vi "Final_Simulator_Run.vi"(7 "Mass Flow (lbm/min) vs. Pressure Drop (inH2O) - Real Data":dbl[][](array[numeric])=[[0.5, 0.015], [1.0, 0.062], [1.5, 0.141], [2.0, 0.252], [2.5, 0.395], [3.5, 0.778]], 8 "error in (no error)":errorcluster, 9 "Tuners":T1={"Inlet Diameter (in)"=0.0, "Outlet Diameter (in)"=0.0, " Length (in)"=0.0, "   Diameter (in)"=0.0, "D_h (in)"=0.0, "OAR"=0.95, "Run Optimizer"=FALSE} {"OAR" items=["0.92"=0.92, "0.93"=0.93, "0.94"=0.94, "0.95"=0.95, "0.96"=0.96]; "D_h (in)" items=["0.0625"=0.0625, "0.125"=0.125, "0.250"=0.25]; "Diameter (in)" min=0.1 max=6.0 scale=0.0..6.0 scale format="%#_3g"; "Length (in)" min=0.1 max=5.0 scale=0.0..6.0 scale format="%#_3g"; "Outlet Diameter (in)" min=0.1 max=5.0 scale=0.0..5.0 scale format="%#_3g"; "Inlet Diameter (in)" min=0.1 max=5.0 scale=0.0..5.0}, 10 "System Configuration":T2={"P_amb (psia)"=0.125, "T_in (Deg F)"=14.7, "R_air (ft*lbf)/(lbm*R)"=530.0, "g_c (lbm*ft)/(lbf*s^2)"=53.35, "specific heat ratio"=32.17, "Viscousity (lbm)/(ft*s)"=1.4, "Cd"=0.95, "Mass Flow (lbm/min) vs. Pressure Drop (inH2O) - Real Data"=[[0.5, 0.015], [1.0, 0.062], [1.5, 0.141], [2.0, 0.252], [2.5, 0.395], [3.5, 0.778]]} {"Mass Flow (lbm/min) vs. Pressure Drop (inH2O) - Real Data" format="%_3g"; "P_amb (psia)" format="%#_4g"}, 11 "d_in_guess":dbl) -> (0 "error out":errorcluster, 1 "Flow Type Name":string="Laminar", 2 "Flow Type":u32(colorbox)=6618880, 3 "total_dp_inh2o":dbl[](array[numeric]))   [LabVIEW 2025]
uses:
  controls/Constants.ctl
  controls/Tuners.ctl
panel:
  # "Honeycomb Parameters"
  # "Orifice Parameters"
  # "Pipe Parameters"
  # "AIRFLOW SIMULATOR"
  # "Mass_flowrate"
  # "Pipe_Diameter"
  # "Outlet_Diameter"
  # "Inlet_Diameter"
  # "Honeycomb_Length"
  # "Empirical Flow Path Data"
  # "Mass Flow\n (lbm/min)"
  # "Pressure Drop \n    (inH2O)"
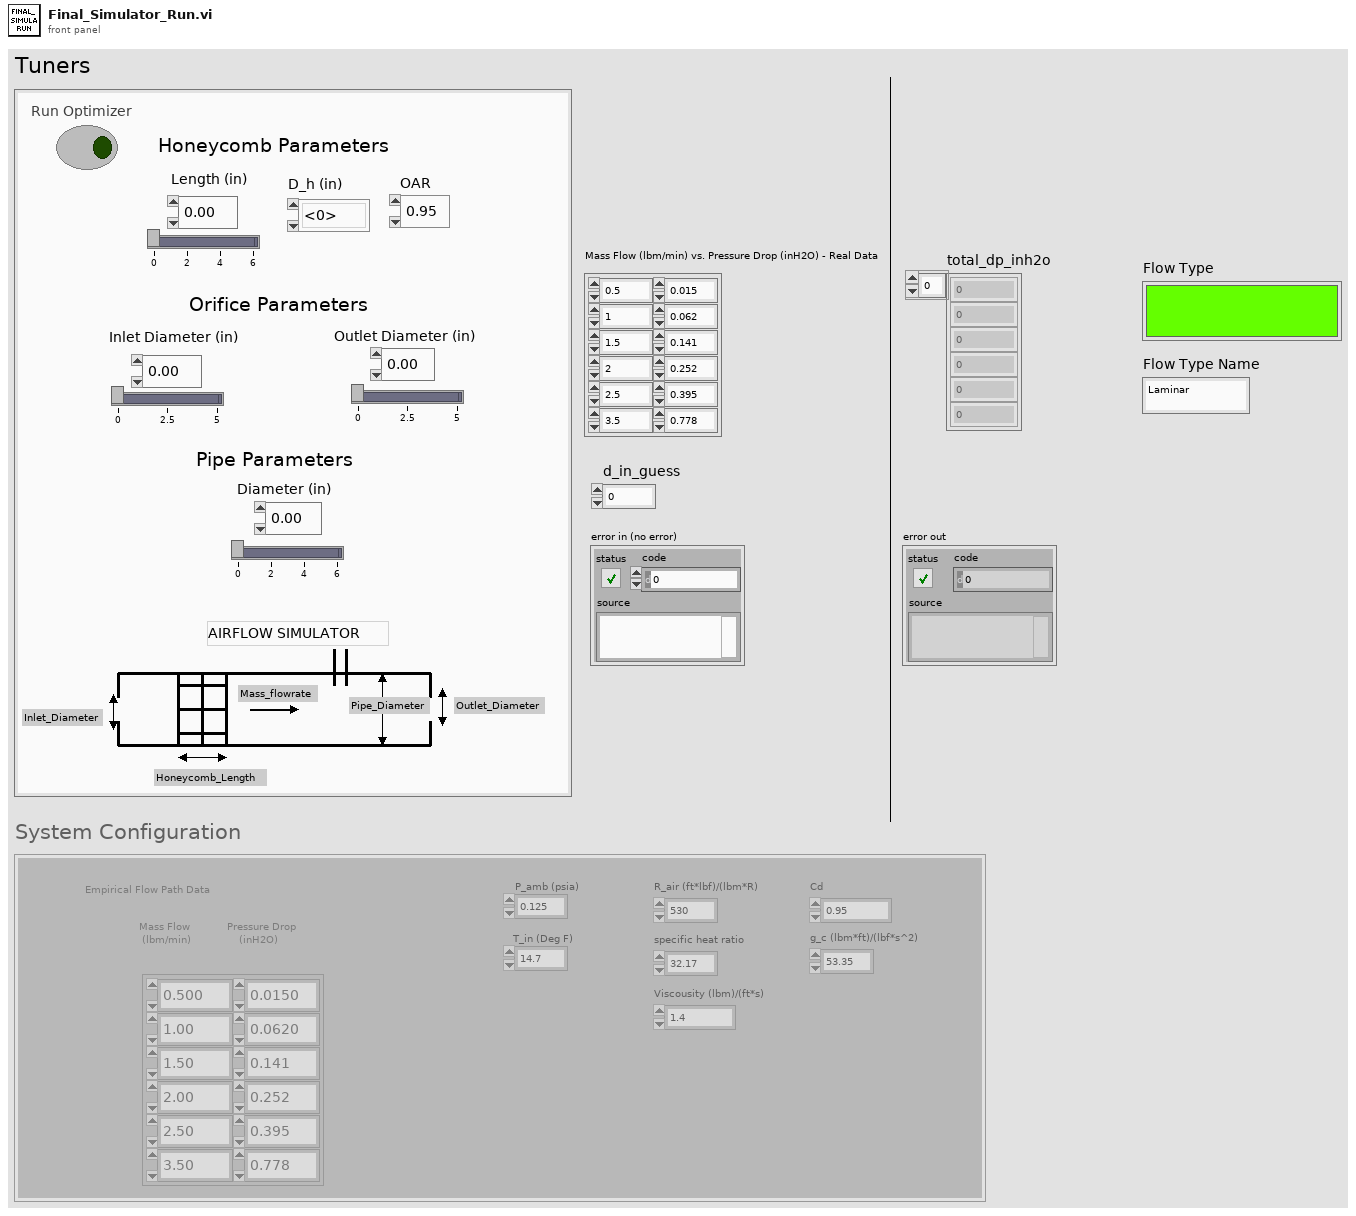
[diagram p1: front panel]
types:
  T1 = typedef "Tuners.ctl" = cluster{"Inlet Diameter (in)":dbl, "Outlet Diameter (in)":dbl, " Length (in)":dbl, "   Diameter (in)":dbl, "D_h (in)":dbl, "OAR":dbl, "Run Optimizer":bool}
  T2 = typedef "Constants.ctl" = cluster{"P_amb (psia)":dbl, "T_in (Deg F)":dbl, "R_air (ft*lbf)/(lbm*R)":dbl, "g_c (lbm*ft)/(lbf*s^2)":dbl, "specific heat ratio":dbl, "Viscousity (lbm)/(ft*s)":dbl, "Cd":dbl, "Mass Flow (lbm/min) vs. Pressure Drop (inH2O) - Real Data":dbl[][]}
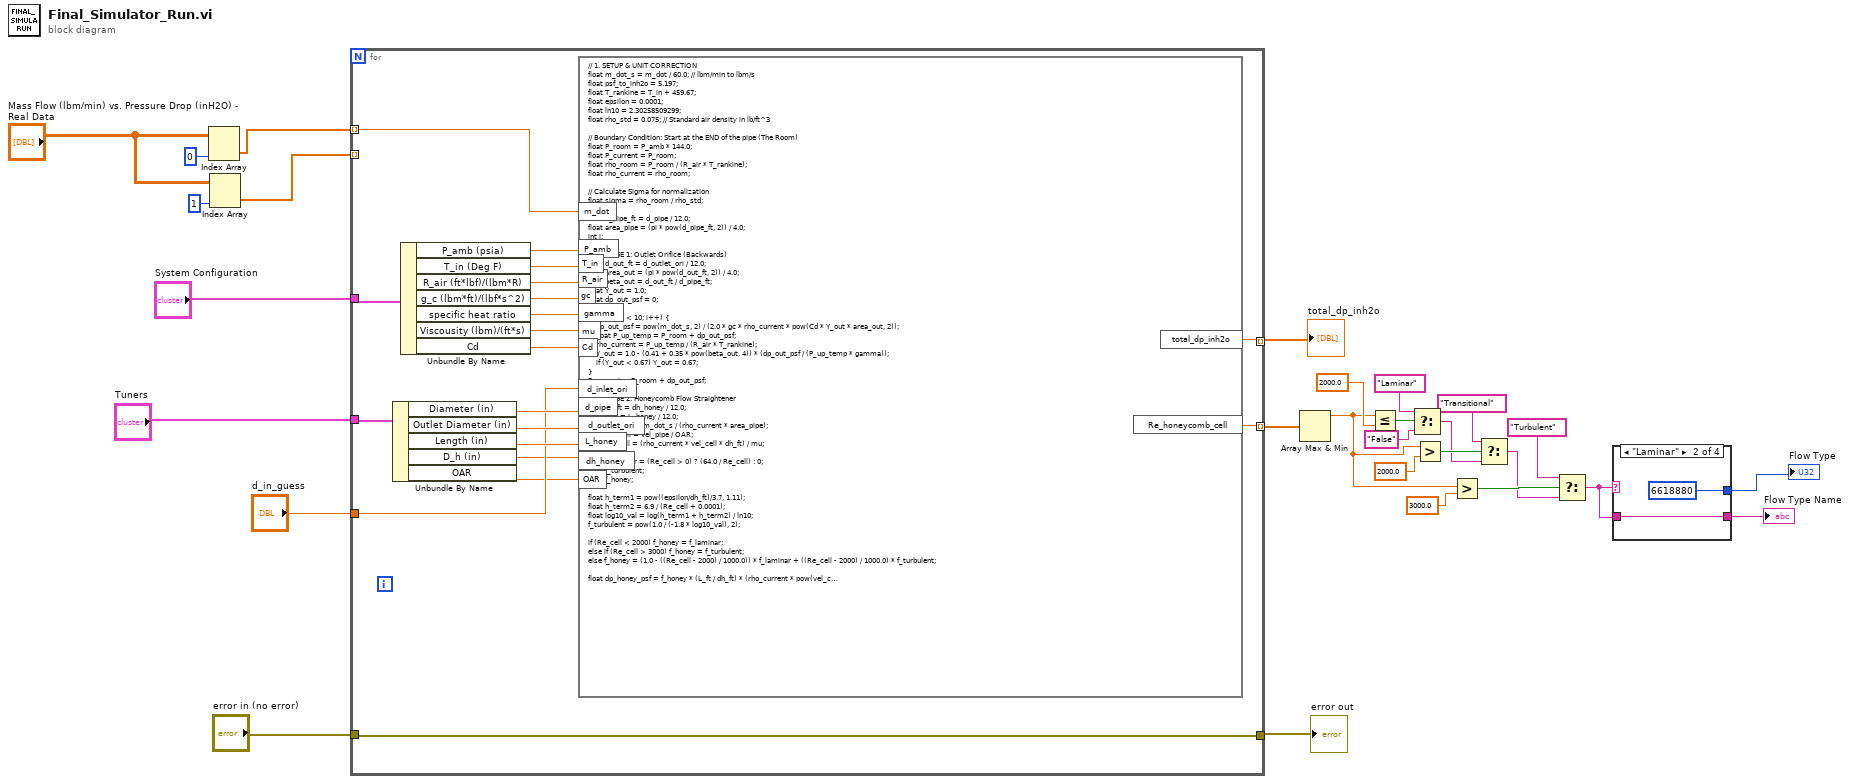
[diagram p0: block diagram]
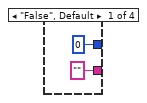
[diagram p2: hidden frame]
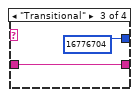
[diagram p3: hidden frame]
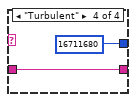
[diagram p4: hidden frame]
diagram:
  n1 = Index Array(array="Mass Flow (lbm/min) vs. Pressure Drop (inH2O) - Real Data", index (col)=0) -> (element=w21:dbl[])  [unwired: 1 in]
  n2 = Index Array(array="Mass Flow (lbm/min) vs. Pressure Drop (inH2O) - Real Data", index (col)=1) -> (element=w20:dbl[])  [unwired: 1 in]
  n3 = for {
    tunnel: "Tuners" -> [w47]
    tunnel: "System Configuration" -> [w45]
    tunnel: [w36] -> w26
    tunnel: "error in (no error)" -> [w36]
    tunnel: [w35] -> w28 mode=indexing
    tunnel: [w34] -> w17 mode=indexing
    tunnel: w20 -> [_] mode=indexing
    tunnel: "d_in_guess" -> [w32]
    tunnel: w21 -> [w31] mode=indexing
    n4 = Unbundle By Name(w47) -> ("Diameter (in)"=w46:dbl, "Outlet Diameter (in)"=w41:dbl, "Length (in)"=w40:dbl, "D_h (in)"=w30:dbl, "OAR"=w29:dbl)
    n5 = Unbundle By Name(w45) -> ("P_amb (psia)"=w44:dbl, "T_in (Deg F)"=w37:dbl, "R_air (ft*lbf)/(lbm*R)"=w38:dbl, "g_c (lbm*ft)/(lbf*s^2)"=w39:dbl, "specific heat ratio"=w43:dbl, "Viscousity (lbm)/(ft*s)"=w42:dbl, "Cd"=w33:dbl)
    n6 = formula code="// 1. SETUP & UNIT CORRECTION\nfloat m_dot_s = m_dot / 60.0; // lbm/min to lbm/s\nfloat psf_to_inh2o = 5.197;\nfloat T_rankine = T_in + 459.67; \nfloat epsilon = 0.0001; \nfloat ln10 = 2.30258509299; \nfloat rho_std = 0.075; // Standard air density in lb/ft^3\n\n// Boundary Condition: Start at the END of the pipe (The Room)\nfloat P_room = P_amb * 144.0; \nfloat P_current = P_room;\nfloat rho_room = P_room / (R_air * T_rankine); \nfloat rho_current = rho_room;\n\n// Calculate Sigma for normalization\nfloat sigma = rho_room / rho_std;\n\nfloat d_pipe_ft = d_pipe / 12.0;\nfloat area_pipe = (pi * pow(d_pipe_ft, 2)) / 4.0;\nint i;\n\n// 2. STAGE 1: Outlet Orifice (Backwards)\nfloat d_out_ft = d_outlet_ori / 12.0;\nfloat area_out = (pi * pow(d_out_ft, 2)) / 4.0;\nfloat beta_out = d_out_ft / d_pipe_ft;\nfloat Y_out = 1.0;\nfloat dp_out_psf = 0;\n\nfor (i = 0; i < 10; i++) {\n    dp_out_psf = pow(m_dot_s, 2) / (2.0 * gc * rho_current * pow(Cd * Y_out * area_out, 2));\n    float P_up_temp = P_room + dp_out_psf;\n    rho_current = P_up_temp / (R_air * T_rankine);\n    Y_out = 1.0 - (0.41 + 0.35 * pow(beta_out, 4)) * (dp_out_psf / (P_up_temp * gamma));\n    if (Y_out < 0.67) Y_out = 0.67;\n}\nP_current = P_room + dp_out_psf;\n\n// 3. STAGE 2: Honeycomb Flow Straightener\nfloat dh_ft = dh_honey / 12.0;\nfloat L_ft = L_honey / 12.0; \nfloat vel_pipe = m_dot_s / (rho_current * area_pipe);\nfloat vel_cell = vel_pipe / OAR; \nfloat Re_cell = (rho_current * vel_cell * dh_ft) / mu; \n\nfloat f_laminar = (Re_cell > 0) ? (64.0 / Re_cell) : 0;\nfloat f_turbulent;\nfloat f_honey;\n\nfloat h_term1 = pow((epsilon/dh_ft)/3.7, 1.11);\nfloat h_term2 = 6.9 / (Re_cell + 0.0001);\nfloat log10_val = log(h_term1 + h_term2) / ln10; \nf_turbulent = pow(1.0 / (-1.8 * log10_val), 2);\n\nif (Re_cell < 2000) f_honey = f_laminar;\nelse if (Re_cell > 3000) f_honey = f_turbulent;\nelse f_honey = (1.0 - ((Re_cell - 2000) / 1000.0)) * f_laminar + ((Re_cell - 2000) / 1000.0) * f_turbulent;\n\nfloat dp_honey_psf = f_honey * (L_ft / dh_ft) * (rho_current * pow(vel_cell, 2)) / (2.0 * gc);\nP_current += dp_honey_psf;\nrho_current = P_current / (R_air * T_rankine);\n\n// 4. STAGE 3: Inlet Orifice\nfloat d_in_ft = d_inlet_ori / 12.0;\nfloat area_in = (pi * pow(d_in_ft, 2)) / 4.0;\nfloat beta_in = d_in_ft / d_pipe_ft;\nfloat Y_in = 1.0;\nfloat dp_in_psf = 0;\n\nfor (i = 0; i < 10; i++) {\n    dp_in_psf = pow(m_dot_s, 2) / (2.0 * gc * rho_current * pow(Cd * Y_in * area_in, 2));\n    float P_up_temp = P_current + dp_in_psf;\n    rho_current = P_up_temp / (R_air * T_rankine);\n    Y_in = 1.0 - (0.41 + 0.35 * pow(beta_in, 4)) * (dp_in_psf / (P_up_temp * gamma));\n    if (Y_in < 0.67) Y_in = 0.67;\n}\nP_current += dp_in_psf;\n\n// 5. FINAL OUTPUTS (Standardized to Sigma-dP)\nfloat raw_total_dp_inh2o = (P_current - P_room) / psf_to_inh2o;\ntotal_dp_inh2o = raw_total_dp_inh2o * sigma; // This is now Sigma Delta Pressure\nRe_honeycomb_cell = Re_cell;"("d_inlet_ori"=w32, "d_pipe"=w46, "gamma"=w43, "P_amb"=w44, "m_dot"=w31, "OAR"=w29, "mu"=w42, "d_outlet_ori"=w41, "L_honey"=w40, "gc"=w39, "R_air"=w38, "T_in"=w37, "dh_honey"=w30, "Cd"=w33) -> ("total_dp_inh2o"=w35:dbl, "Re_honeycomb_cell"=w34:dbl)
  }
  "total_dp_inh2o" <- w28
  "error out" <- w26
  n7 = Array Max & Min(array=w17) -> (max value=w4:dbl)  [unwired: 3 out]
  n8 = Less Or Equal?(x=w4, y=2000.0) -> (x <= y?=w16:bool)
  n9 = Select(t="Laminar", s=w16, f="False") -> (s? t:f=w11:string)
  n10 = Greater?(x=w4, y=2000.0) -> (0:w12:bool)
  n11 = Greater?(x=w4, y=3000.0) -> (0:w9:bool)
  n12 = Select(t="Transitional", s=w12, f=w11) -> (s? t:f=w7:string)
  n13 = Select(t="Turbulent", s=w9, f=w7) -> (s? t:f=w3:string)
  n14 = case shown="\"Laminar\"" w3 {
    tunnel: [u32 0 u32 6618880 u32 16776704 u32 16711680] -> w2
    tunnel: ["" ("f") w50 w52 w54] -> w1
    tunnel: w3 -> [_ w50 w52 w54]
    frame "False", Default {
    }
    frame "Laminar" {
    }
    frame "Transitional" {
    }
    frame "Turbulent" {
    }
  }
  "Flow Type Name" <- w1
  "Flow Type" <- w2
